vi "SaveFile.vi"(9 "数据":string[][](array[string]), 10 "文件头":string[](array[string]), 11 "文件路径":path) -> (3 "Success":bool)   [LabVIEW 2011]
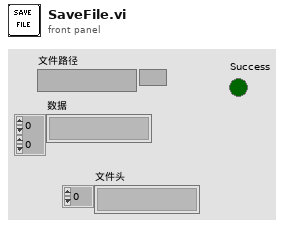
[diagram p1: front panel]
types:
  T1 = enum16{"open", "replace", "create", "open or create", "replace or create", "replace or create with confirmation"}
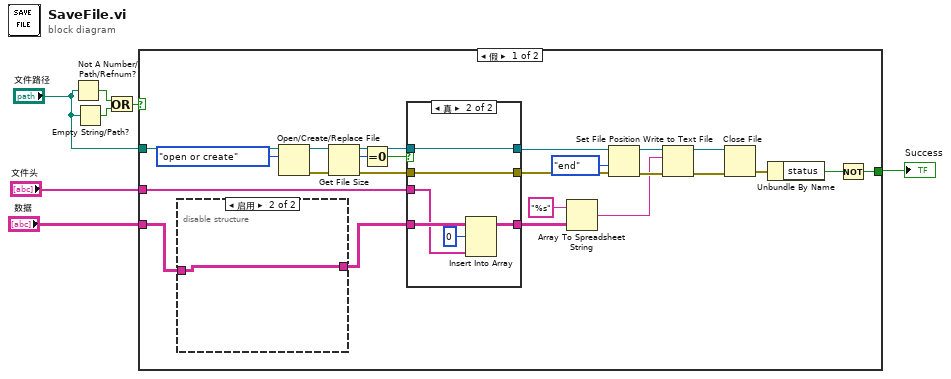
[diagram p0: block diagram]
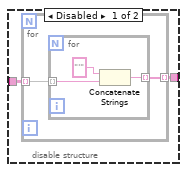
[diagram p2: hidden frame]
diagram:
  n1 = Not A Number/Path/Refnum?(number/path/refnum="文件路径") -> (NaN/Path/Refnum?=w7:bool)
  n2 = Empty String/Path?(string/path="文件路径") -> (empty?=w6:bool)
  n3 = Or(x=w7, y=w6) -> (x .or. y?=w5:bool)
  n4 = case shown="假" w5 {
    tunnel: "文件路径" -> [w31 _]
    tunnel: "文件头" -> [w23 _]
    tunnel: "数据" -> [w22 _]
    tunnel: [w8 _] -> w1
    frame False {
      n5 = disable-structure shown="启用" {
        disable-tunnel: w22 -> [w33 w39]
        disable-tunnel: [w32 w39] -> w21
        frame Disabled {
          n6 = for {
            tunnel: w33 -> [w35] mode=indexing
            tunnel: [w34] -> w32 mode=indexing
            n7 = for {
              tunnel: w35 -> [w38] mode=indexing
              tunnel: [w36] -> w34 mode=indexing
              n8 = Concatenate Strings("'" ("字符串"), w38) -> (w36:string)
            }
          }
        }
        frame Enabled {
        }
      }
      n9 = Open/Create/Replace File(file path (use dialog)=w31, operation (0:open)=T1."open or create" ("操作(0:open)")) -> (refnum out=w29:refnum<file>, error out=w28:errorcluster)  [unwired: 4 in, 1 out]
      n10 = Get File Size(file=w29, error in=w28) -> (refnum out=w25:refnum<file>, size (in bytes)=w27:i64, 0:w24:errorcluster)
      n11 = Equal To 0?(x=w27) -> (x = 0?=w26:bool)
      n12 = case shown="真" w26 {
        tunnel: w25 -> [w41 w44]
        tunnel: w24 -> [w40 w43]
        tunnel: w23 -> [_ w47]
        tunnel: w21 -> [w42 w48]
        tunnel: [w42 w45] -> w19
        tunnel: [w41 w44] -> w18
        tunnel: [w40 w43] -> w17
        frame False {
        }
        frame True {
          n13 = Insert Into Array(array=w48, index (row)=0 ("索引 (行)"), new element=w47) -> (w45:string[][])  [unwired: 1 in]
        }
      }
      n14 = Array To Spreadsheet String(array=w19, 3:"%s" ("格式字符串")) -> (spreadsheet string=w13:string)  [unwired: 1 in]
      n15 = Set File Position(refnum=w18, from (0:start)=enum16{"start", "end", "current"}."end" ("自（0:起始）"), error in=w17) -> (refnum out=w15:refnum<file>, error out=w14:errorcluster)  [unwired: 1 in]
      n16 = Write to Text File(file (use dialog)=w15, text=w13, error in=w14) -> (refnum out=w11:refnum<file>, error out=w12:errorcluster)  [unwired: 1 in, 1 out]
      n17 = Close File(refnum=w11, error in=w12) -> (error out=w10:errorcluster)  [unwired: 1 out]
      n18 = Unbundle By Name(w10) -> ("status"=w9:bool)
      n19 = Not(x=w9) -> (.not. x?=w8:bool)
    }
    frame True {
    }
  }
  "Success" <- w1
